vi "GlobalFullBin.vi"() -> ()   [LabVIEW 2010]
panel:
  out "Full":bool
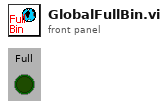
[diagram p1: front panel]
diagram:
